vi "Tactile Controller v1.3.vi"() -> ()   [LabVIEW 2013]
uses:
  <vilib>/Instr/_visa.llb/VISA Configure Serial Port (Instr).vi
panel:
  in  "Refresh":bool
  in  "Switch":bool
  in  "Comm":bool
  out "Message Board":string
  in  "Serial Port":refnum<visa-resource-name>="COM7"
  in  "stop":bool
  out "read buffer":string
  in  "Trials":dbl=200.0
  in  "Inter-Stimulus Interval":dbl=1200.0
  in  "Vibro cycles":dbl=20.0
  in  "Jitter":dbl=100.0
  in  "Pin up duration":dbl=5.0
  in  "Stimuli Type":T1(ring)=enum."Steady State"
  in  "Cell5":bool=TRUE
  in  "Cell4":bool=TRUE
  in  "Cell3":bool=TRUE
  in  "Cell2":bool=TRUE
  in  "Cell1":bool=TRUE
  in  "SSF5":dbl=11.0
  in  "SSF4":dbl=8.0
  in  "SSF3":dbl=7.0
  in  "SSF2":dbl=5.0
  in  "SSF1":dbl=2.0
  in  "C5P8":bool=TRUE
  in  "C5P7":bool=TRUE
  in  "C5P6":bool=TRUE
  in  "C5P5":bool=TRUE
  in  "C5P4":bool=TRUE
  in  "C5P3":bool=TRUE
  in  "C5P2":bool=TRUE
  in  "C5P1":bool=TRUE
  in  "C4P8":bool=TRUE
  in  "C4P7":bool=TRUE
  in  "C4P6":bool=TRUE
  in  "C4P5":bool=TRUE
  in  "C4P4":bool=TRUE
  in  "C4P3":bool=TRUE
  in  "C4P2":bool=TRUE
  in  "C4P1":bool=TRUE
  in  "C3P8":bool=TRUE
  in  "C3P7":bool=TRUE
  in  "C3P6":bool=TRUE
  in  "C3P5":bool=TRUE
  in  "C3P4":bool=TRUE
  in  "C3P3":bool=TRUE
  in  "C3P2":bool=TRUE
  in  "C3P1":bool=TRUE
  in  "C2P8":bool=TRUE
  in  "C2P7":bool=TRUE
  in  "C2P6":bool=TRUE
  in  "C2P5":bool=TRUE
  in  "C2P4":bool=TRUE
  in  "C2P3":bool=TRUE
  in  "C2P2":bool=TRUE
  in  "C2P1":bool=TRUE
  in  "C1P8":bool=TRUE
  in  "C1P7":bool=TRUE
  in  "C1P6":bool=TRUE
  in  "C1P5":bool=TRUE
  in  "C1P4":bool=TRUE
  in  "C1P3":bool=TRUE
  in  "C1P2":bool=TRUE
  in  "C1P1":bool=TRUE
  # "ms"
  # "ms"
  # "ms"
  # "1                           2                         3                        4                         5"
  # "Steady State Frequency [Hz]"
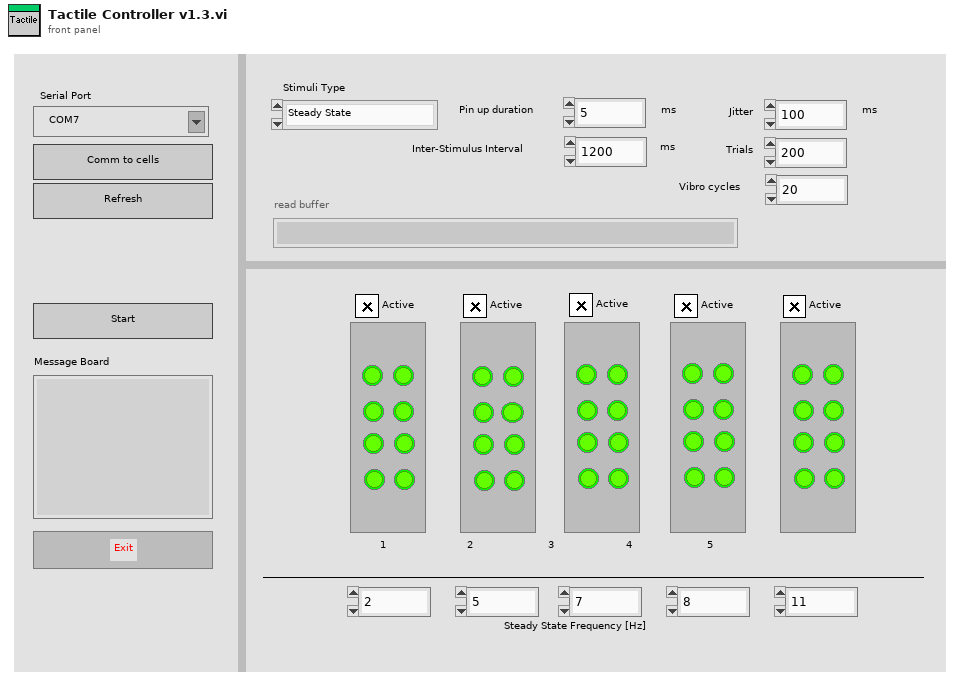
[diagram p1: front panel]
types:
  T1 = enum16{"Transient", "Steady State", "Vibrotactile"}
  T2 = enum8{"Enabled", "Disabled", "Disabled and Grayed Out"}
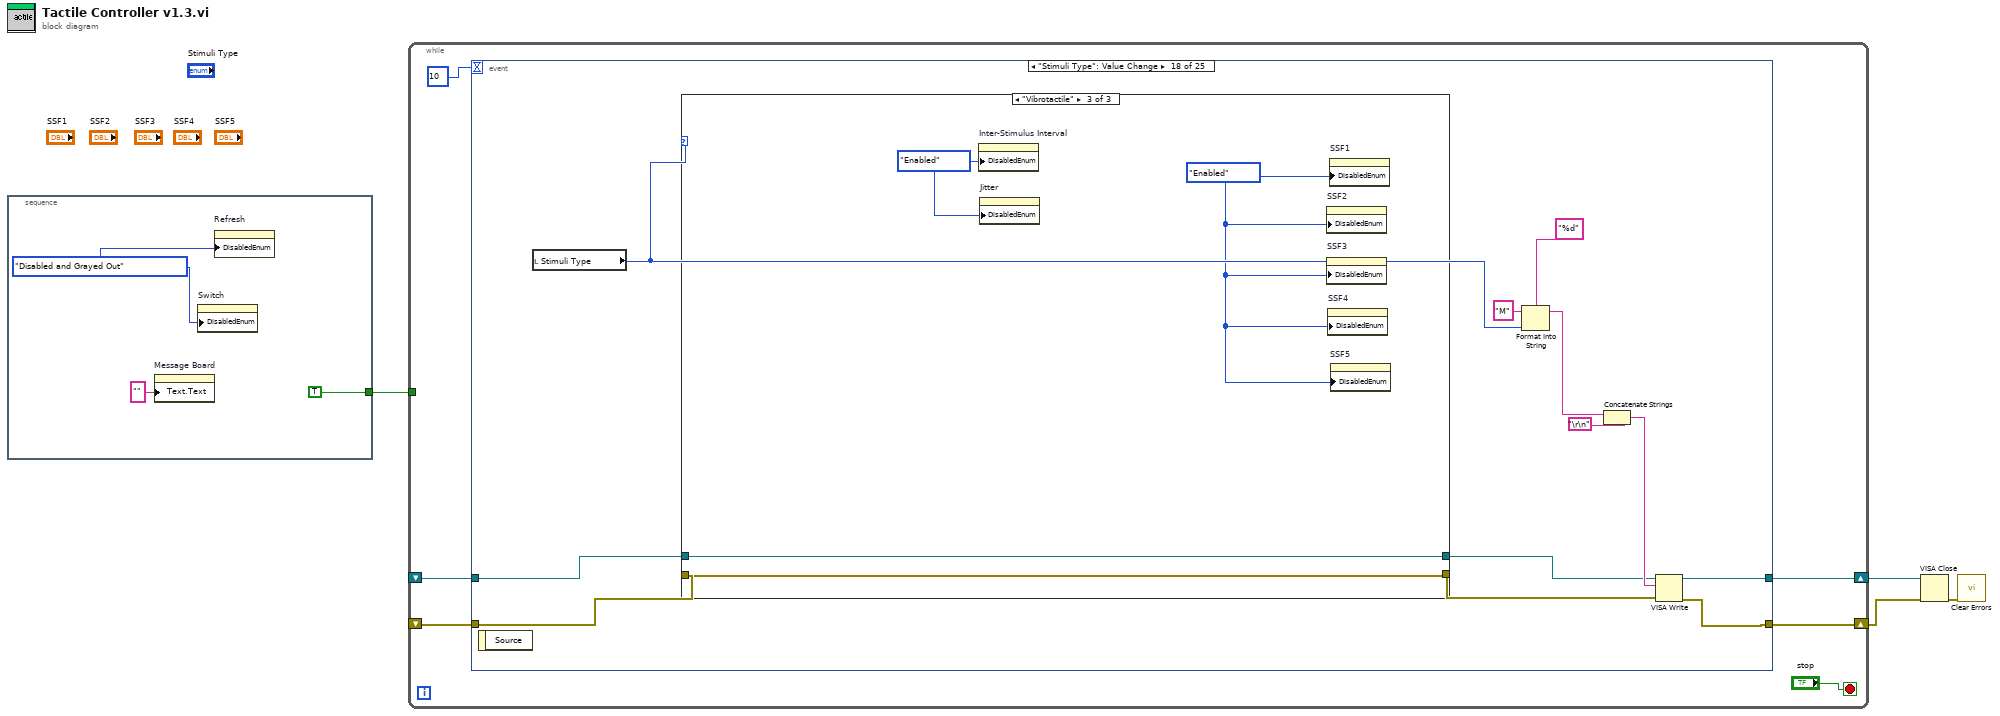
[diagram p0: block diagram]
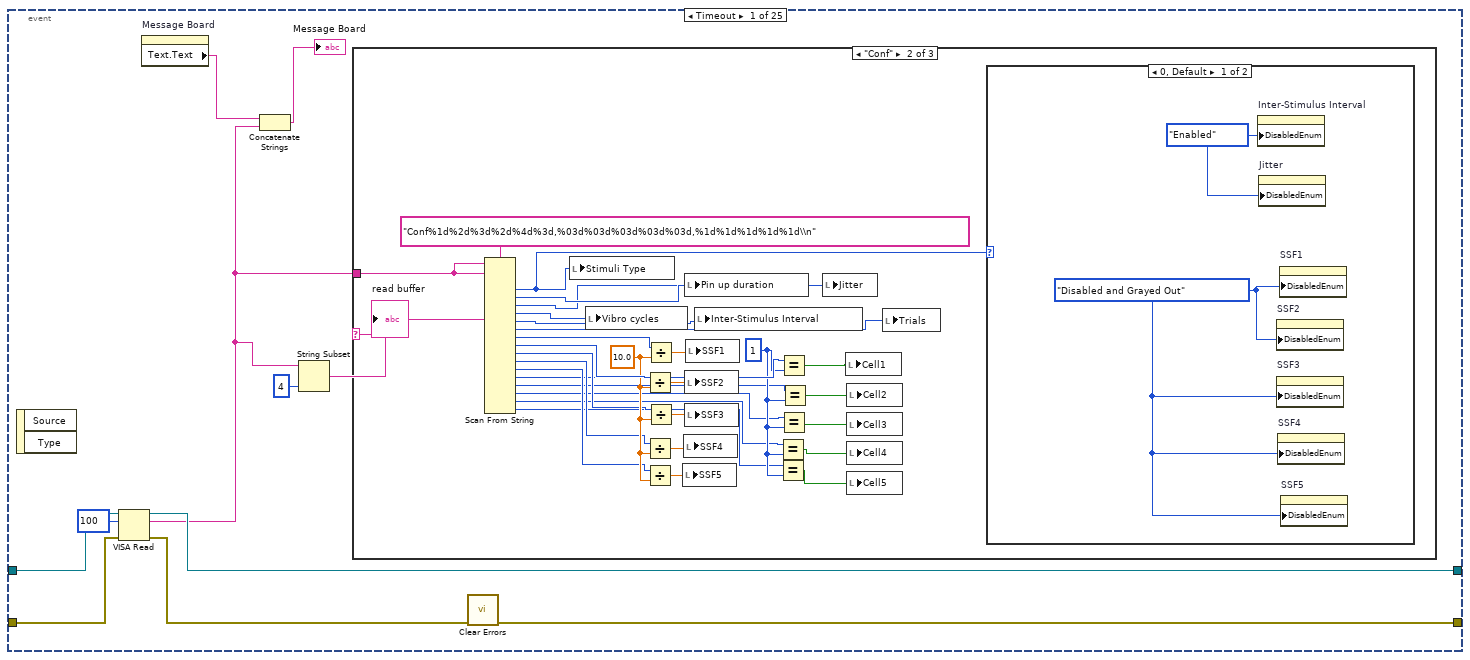
[diagram p2: hidden frame]
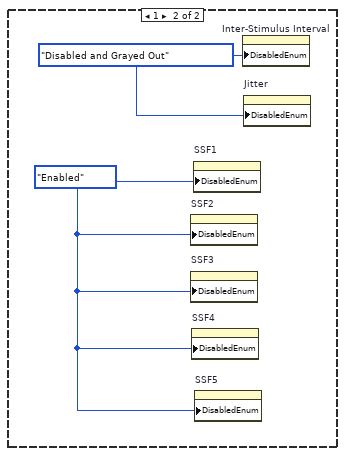
[diagram p4: hidden frame]
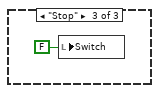
[diagram p5: hidden frame]
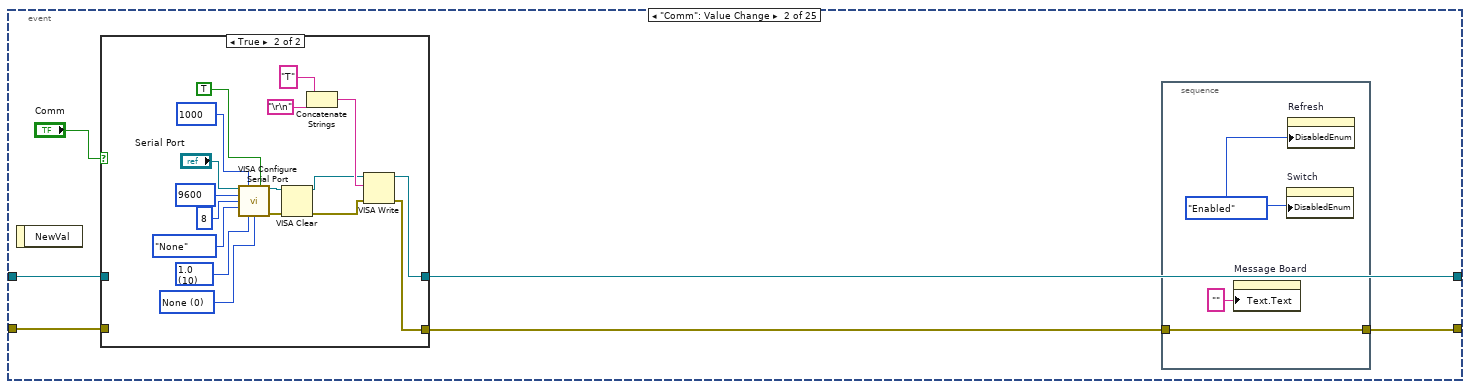
[diagram p6: hidden frame]
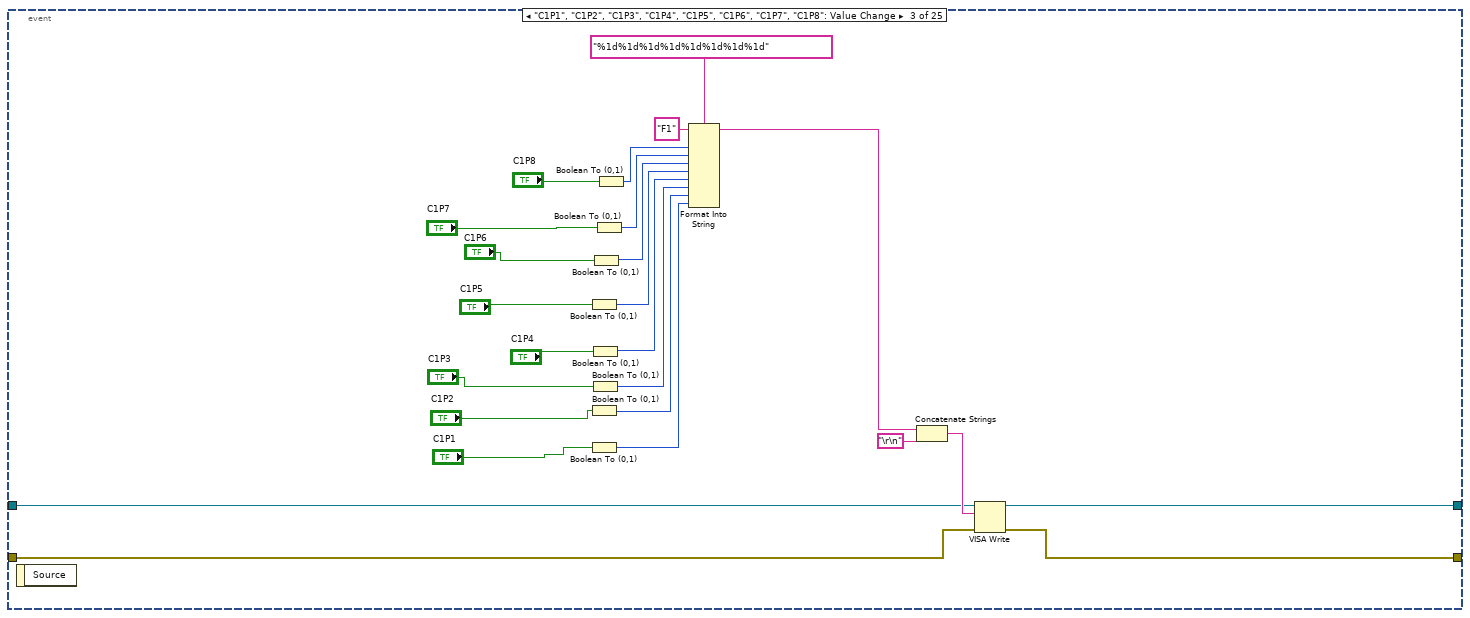
[diagram p8: hidden frame]
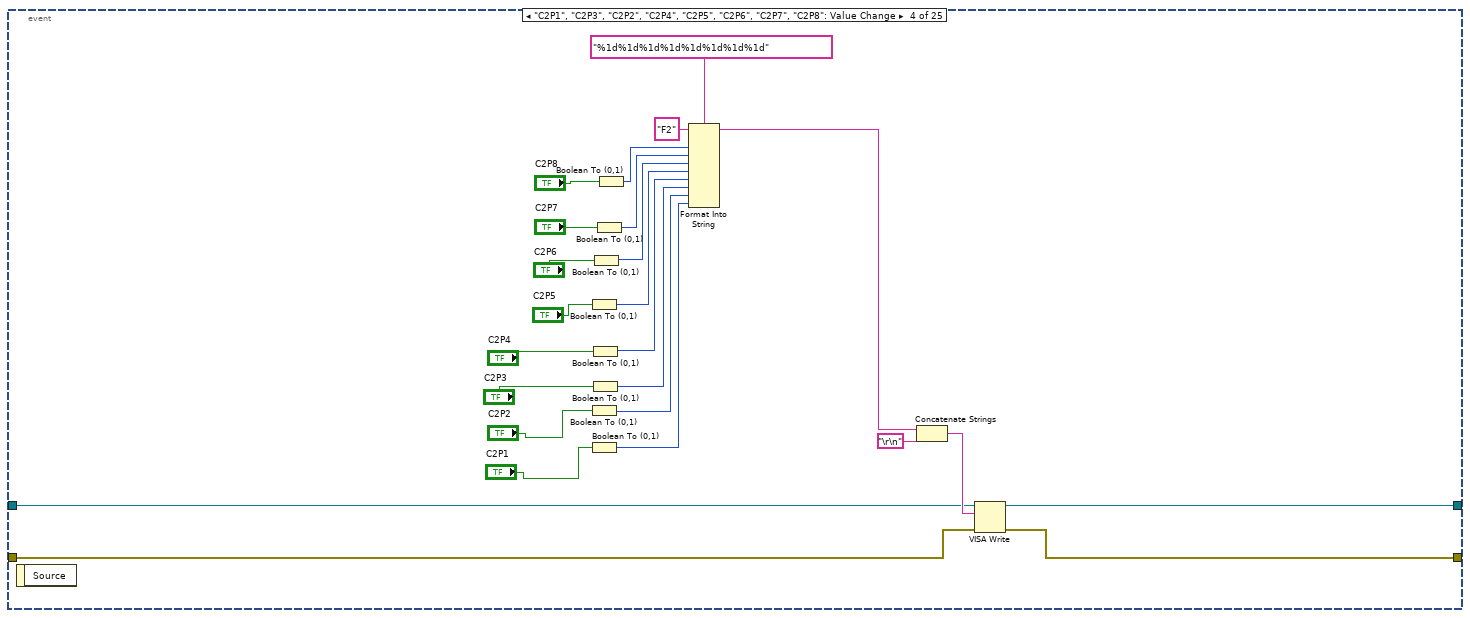
[diagram p9: hidden frame]
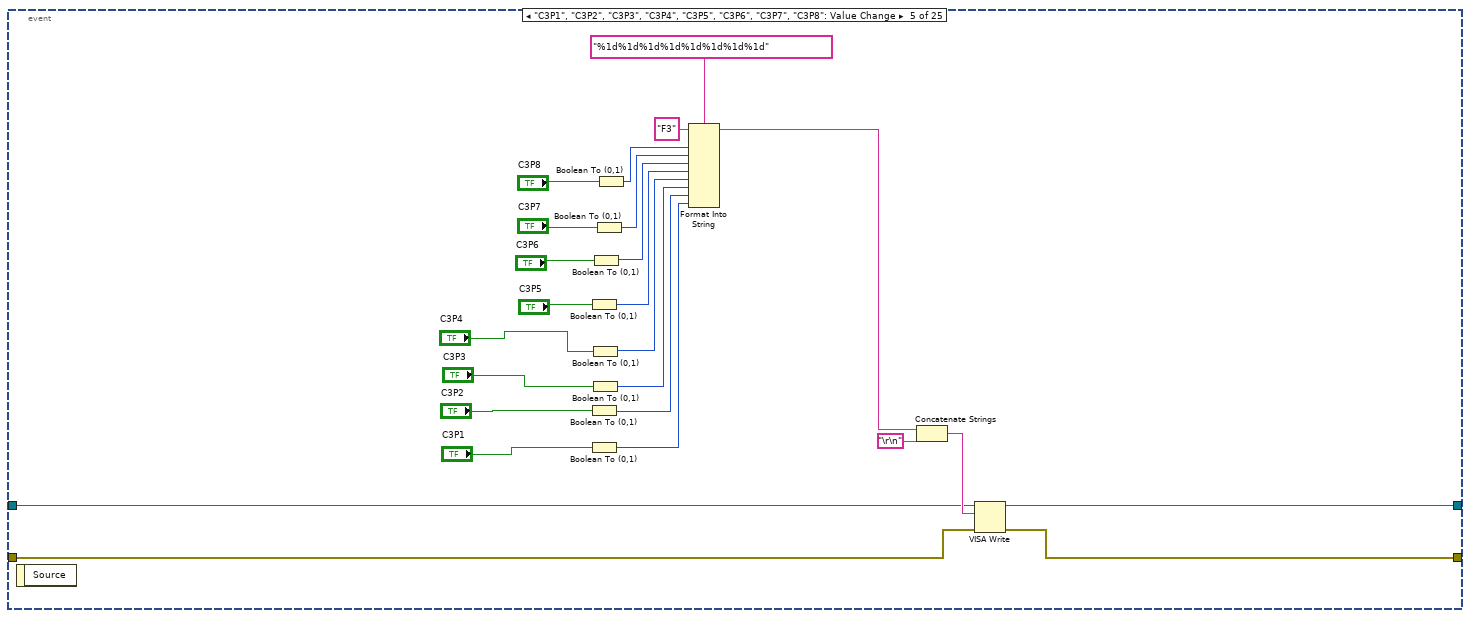
[diagram p10: hidden frame]
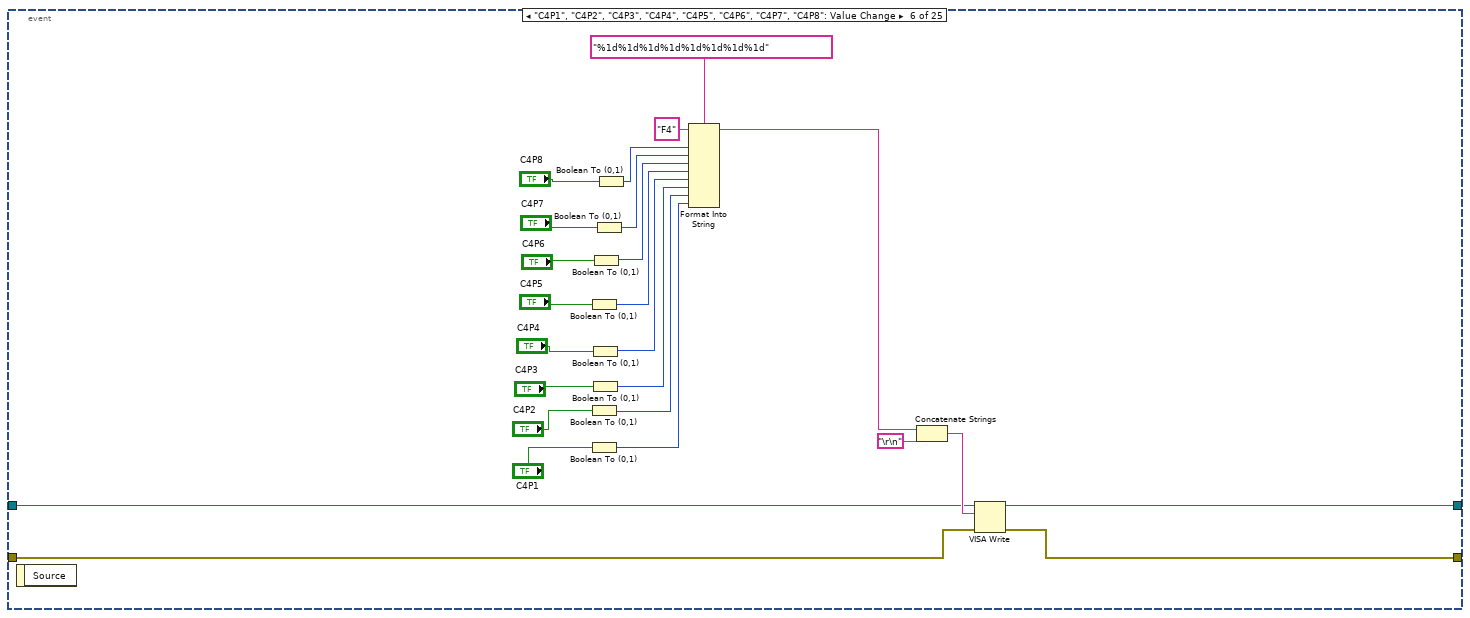
[diagram p11: hidden frame]
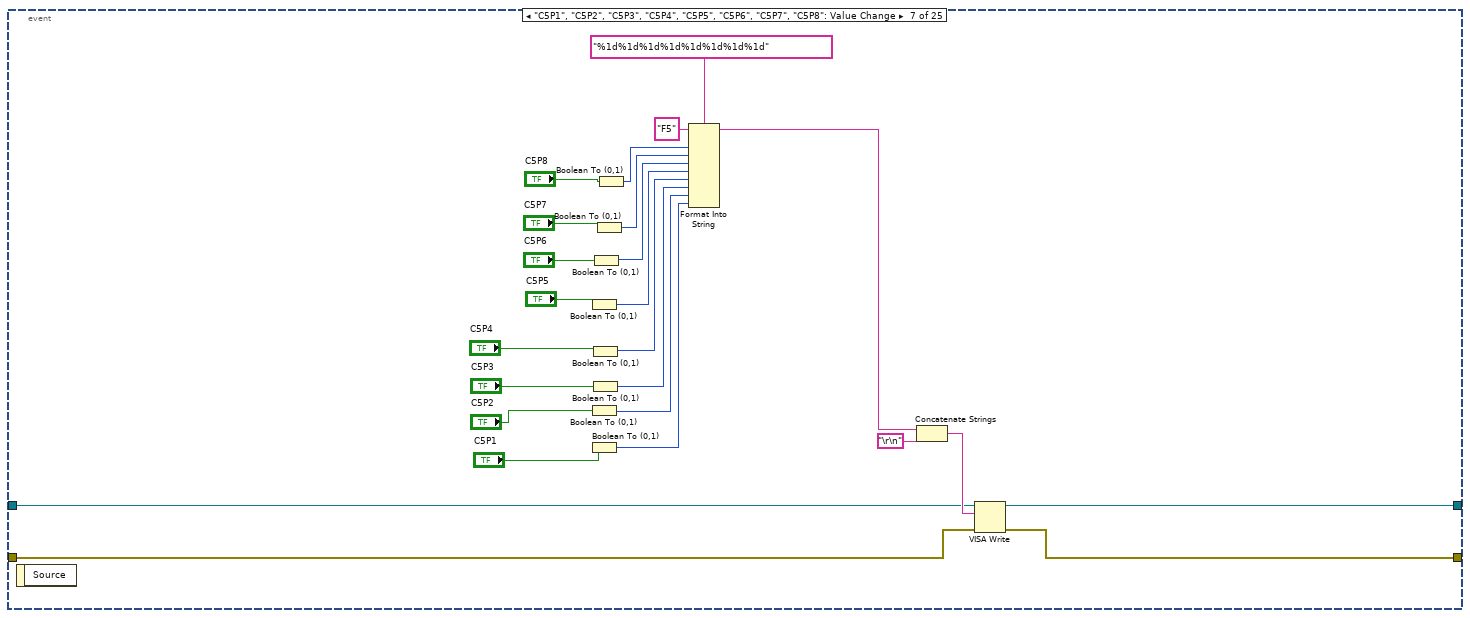
[diagram p12: hidden frame]
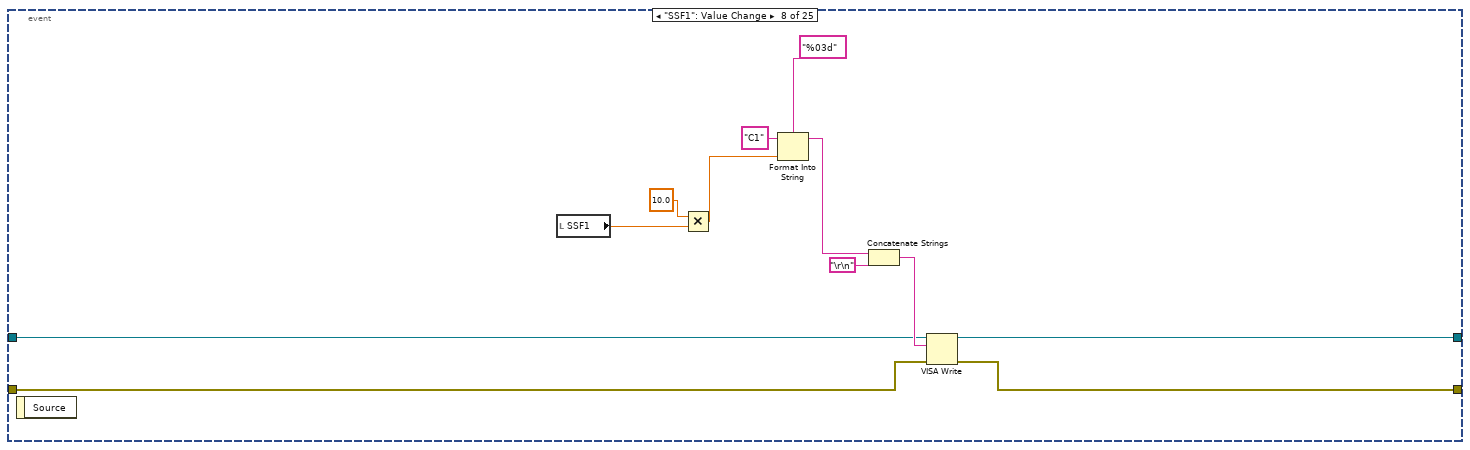
[diagram p13: hidden frame]
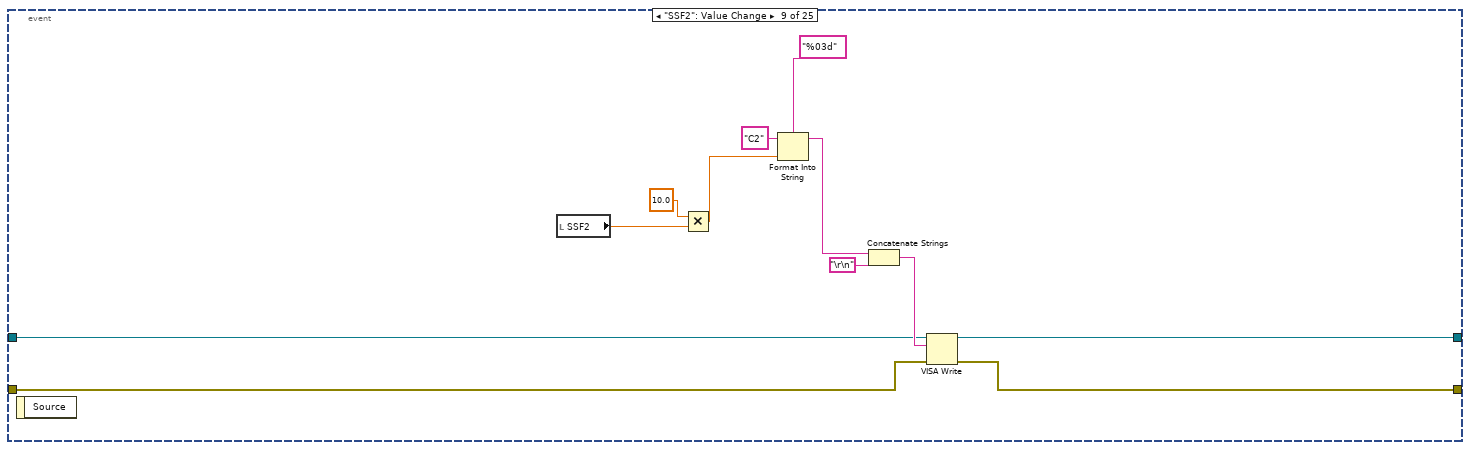
[diagram p14: hidden frame]
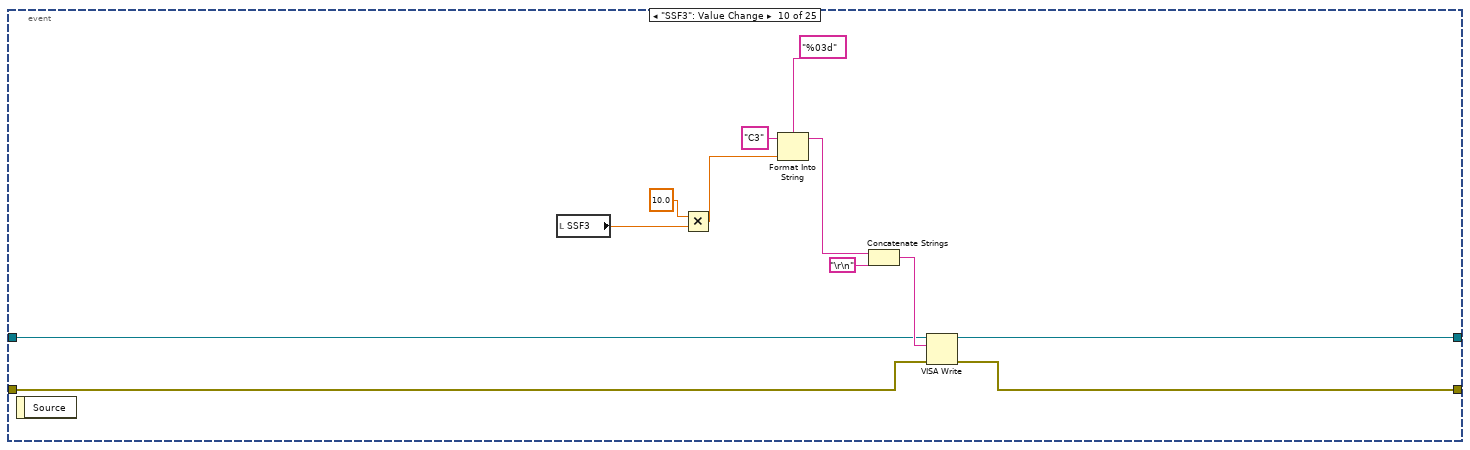
[diagram p15: hidden frame]
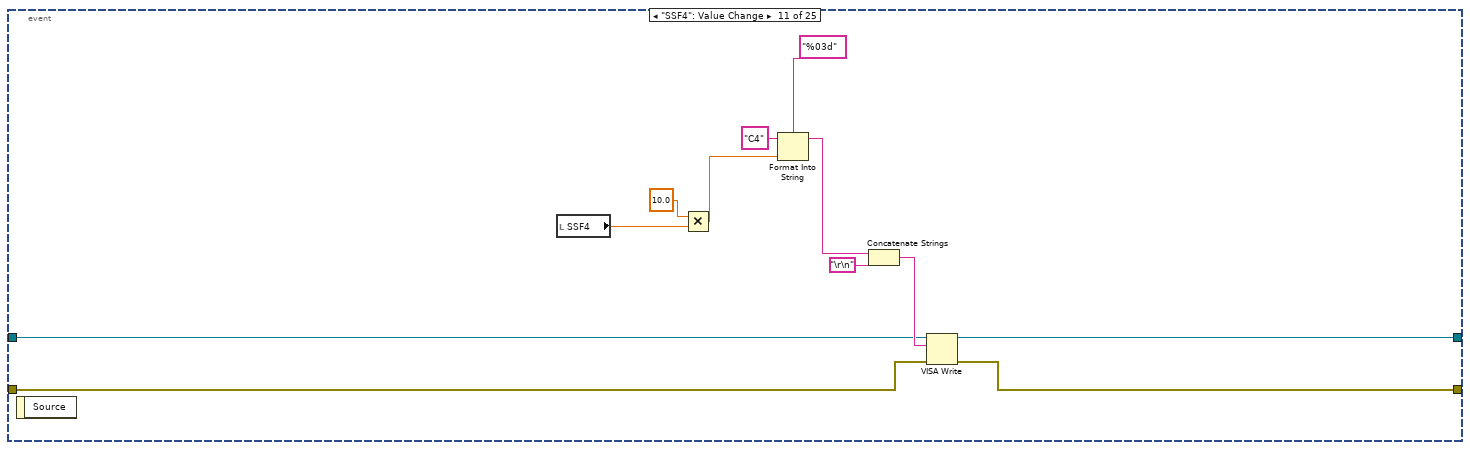
[diagram p16: hidden frame]
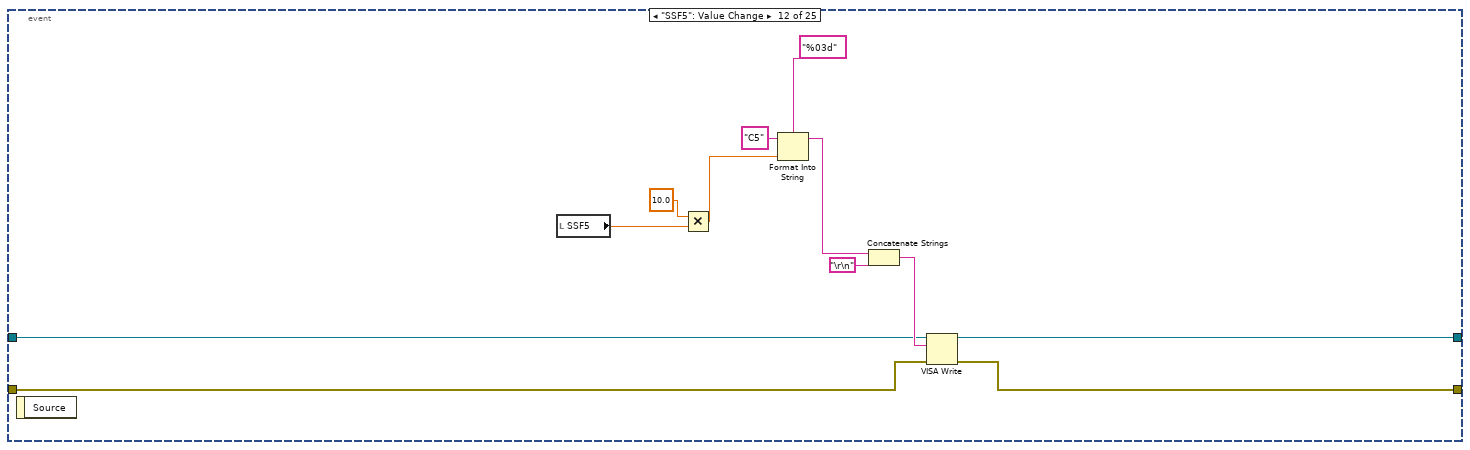
[diagram p17: hidden frame]
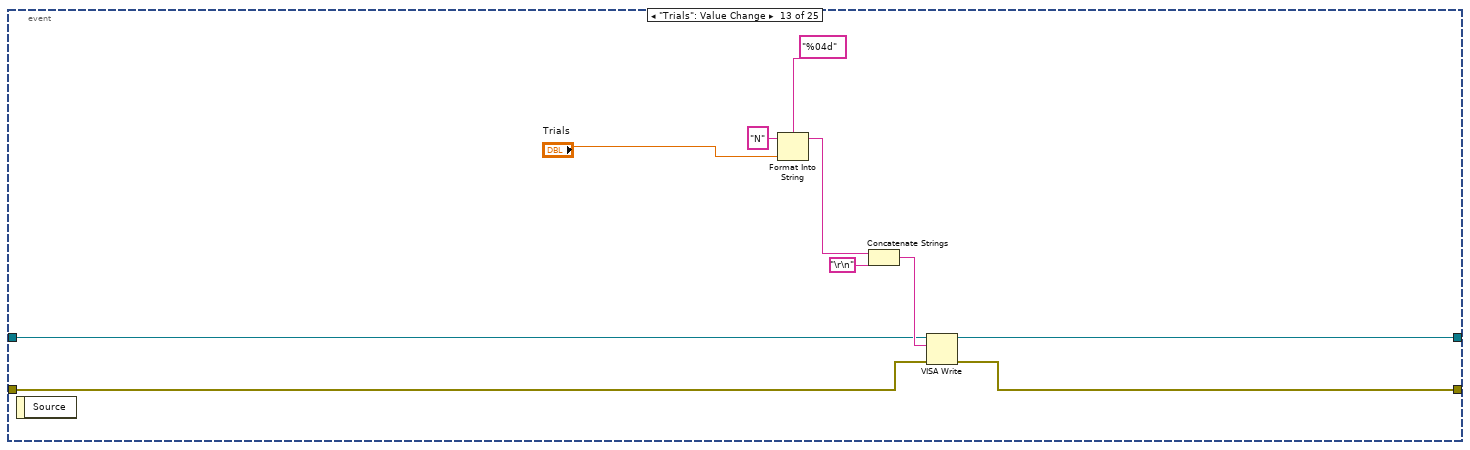
[diagram p18: hidden frame]
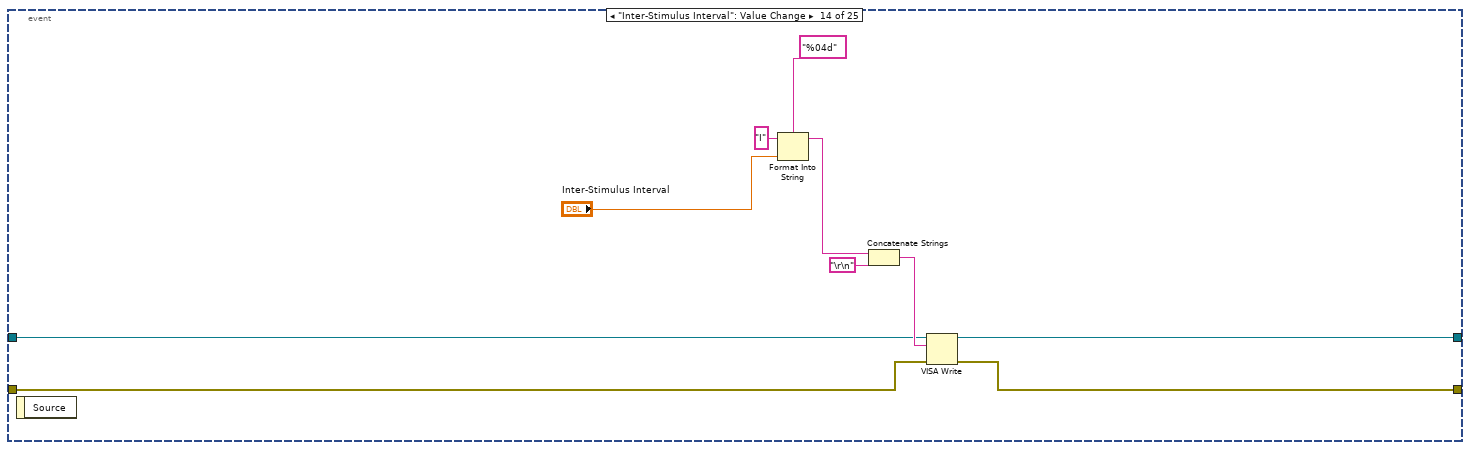
[diagram p19: hidden frame]
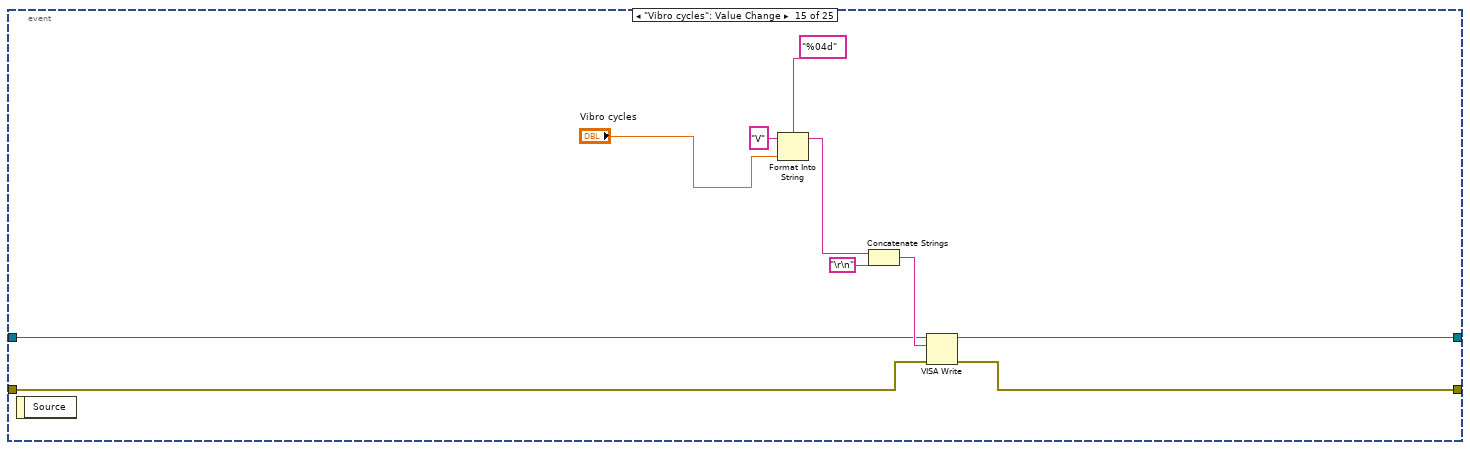
[diagram p20: hidden frame]
diagram:
  n1 = stacked-sequence {
    tunnel: [TRUE] -> w1
    frame #0 {
      w5 = T2."Disabled and Grayed Out" ("Disabled")
      n2 = property on="Message Board" class="Str"("Text.Text"="") -> ()  [unwired: 2 in, 2 out]
      n3 = property on="Switch" class="Bool (strict)"("DisabledEnum"=w5) -> ()  [unwired: 2 in, 2 out]
      n4 = property on="Refresh" class="Bool (strict)"("DisabledEnum"=w5) -> ()  [unwired: 2 in, 2 out]
    }
  }
  n5 = while {
    shift-right: [w11] -> w3
    shift-left: _ -> [w12]
    shift-right: [w8] -> w2
    shift-left: _ -> [w9]
    tunnel: w1 -> [_]
    stop <- "stop" stop-if-true
    n6 = event shown="[17] \"Stimuli Type\": Value Change" {
      selector: _ -> [_ _ _ _ _ _ _ _ _ _ _ _ _ _ _ _ _ _ _ _ _ _ _ _ _]
      dyn-events: _ -> [_ _ _ _ _ _ _ _ _ _ _ _ _ _ _ _ _ _ _ _ _ _ _ _ _]
      timeout: u32 10 ("milliseconds to wait") -> [_ _ _ _ _ _ _ _ _ _ _ _ _ _ _ _ _ _ _ _ _ _ _ _ _]
      tunnel: w12 -> [w22 w64 w98 w123 w148 w173 w198 w218 w230 w242 w254 w266 w276 w286 w296 w306 w316 w333 w349 w361 w372 w383 w394 w406 w423]
      tunnel: [w24 w62 w96 w121 w146 w171 w196 w216 w228 w240 w252 w264 w274 w284 w294 w304 w314 w323 w348 w360 w371 w382 w393 w405 w422] -> w11
      tunnel: w9 -> [w21 w63 w99 w124 w149 w174 w199 w219 w231 w243 w255 w267 w277 w287 w297 w307 w317 w334 w351 w363 w374 w385 w396 w404 w425]
      tunnel: [w20 w60 w97 w122 w147 w172 w197 w217 w229 w241 w253 w265 w275 w285 w295 w305 w315 w325 w347 w359 w370 w381 w392 w403 w424] -> w8
      event Timeout {
        n7 = event-data() -> ()  [unwired: 1 in, 2 out]
        n8 = VISA Read(VISA resource name=w21, byte count=u32 100, error in (no error)=w22) -> (VISA resource name out=w20:refnum<visa-resource-name>, read buffer=w14:string, error out=w19:errorcluster)  [unwired: 1 out]
        n9 = property on="Message Board" class="Str"() -> ("Text.Text"=w17:string)  [unwired: 2 in, 2 out]
        n10 = Concatenate Strings(w17, w14) -> (→"Message Board":string)
        n11 = String Subset(string=w14, length (rest)=4 ("length (rest)")) -> (substring=w15:string)  [unwired: 1 in]
        n12 = case shown="\"Conf\"" w15 {
          tunnel: w14 -> [_ w54 _]
          frame Default {
          }
          frame "Conf" {
            w34 = i8 1 ("y")
            w42 = 10.0 ("y")
            n13 = Scan From String(format string="Conf%1d%2d%3d%2d%4d%3d,%03d%03d%03d%03d%03d,%1d%1d%1d%1d%1d\\n", input string=w54) -> (output 1=w25:i32, output 2=w52:i32, output 3=w51:i32, output 4=w50:i32, output 5=w49:i32, output 6=w48:i32, output 7=w47:i32, output 8=w44:i32, output 9=w41:i32, output 10=w40:i32, output 11=w39:i32, output 12=w36:i32, output 13=w33:i32, output 14=w32:i32, output 15=w31:i32, output 16=w30:i32)  [unwired: 18 in, 3 out]
            n14 = local write "Stimuli Type"(w25) -> ()
            n15 = local write "Vibro cycles"(w50) -> ()
            n16 = Divide(x=w44, y=w42) -> (x/y=w45:dbl)
            n17 = Divide(x=w40, y=w42) -> (x/y=w38:dbl)
            n18 = Divide(x=w39, y=w42) -> (x/y=w37:dbl)
            n19 = Divide(x=w47, y=w42) -> (x/y=w46:dbl)
            n20 = Divide(x=w41, y=w42) -> (x/y=w43:dbl)
            n21 = local write "SSF5"(w37) -> ()
            n22 = local write "SSF4"(w38) -> ()
            n23 = local write "Pin up duration"(w52) -> ()
            n24 = local write "SSF2"(w45) -> ()
            n25 = local write "SSF3"(w43) -> ()
            n26 = local write "SSF1"(w46) -> ()
            n27 = local write "Inter-Stimulus Interval"(w49) -> ()
            n28 = Equal?(x=w31, y=w34) -> (x = y?=w27:bool)
            n29 = Equal?(x=w30, y=w34) -> (x = y?=w26:bool)
            n30 = Equal?(x=w36, y=w34) -> (x = y?=w35:bool)
            n31 = Equal?(x=w32, y=w34) -> (x = y?=w28:bool)
            n32 = Equal?(x=w33, y=w34) -> (x = y?=w29:bool)
            n33 = local write "Jitter"(w51) -> ()
            n34 = local write "Cell1"(w35) -> ()
            n35 = local write "Cell2"(w29) -> ()
            n36 = local write "Cell3"(w28) -> ()
            n37 = local write "Cell4"(w27) -> ()
            n38 = local write "Cell5"(w26) -> ()
            n39 = local write "Trials"(w48) -> ()
            n40 = case shown="0, Default" w25 {
              frame 0, Default {
                w55 = T2."Enabled" ("Disabled")
                w56 = T2."Disabled and Grayed Out" ("Disabled")
                n41 = property on="Inter-Stimulus Interval" class="DigNum (strict)"("DisabledEnum"=w55) -> ()  [unwired: 2 in, 2 out]
                n42 = property on="Jitter" class="DigNum (strict)"("DisabledEnum"=w55) -> ()  [unwired: 2 in, 2 out]
                n43 = property on="SSF2" class="DigNum (strict)"("DisabledEnum"=w56) -> ()  [unwired: 2 in, 2 out]
                n44 = property on="SSF3" class="DigNum (strict)"("DisabledEnum"=w56) -> ()  [unwired: 2 in, 2 out]
                n45 = property on="SSF4" class="DigNum (strict)"("DisabledEnum"=w56) -> ()  [unwired: 2 in, 2 out]
                n46 = property on="SSF1" class="DigNum (strict)"("DisabledEnum"=w56) -> ()  [unwired: 2 in, 2 out]
                n47 = property on="SSF5" class="DigNum (strict)"("DisabledEnum"=w56) -> ()  [unwired: 2 in, 2 out]
              }
              frame 1 {
                w57 = T2."Enabled" ("Disabled")
                w58 = T2."Disabled and Grayed Out" ("Disabled")
                n48 = property on="SSF2" class="DigNum (strict)"("DisabledEnum"=w57) -> ()  [unwired: 2 in, 2 out]
                n49 = property on="SSF3" class="DigNum (strict)"("DisabledEnum"=w57) -> ()  [unwired: 2 in, 2 out]
                n50 = property on="SSF4" class="DigNum (strict)"("DisabledEnum"=w57) -> ()  [unwired: 2 in, 2 out]
                n51 = property on="SSF1" class="DigNum (strict)"("DisabledEnum"=w57) -> ()  [unwired: 2 in, 2 out]
                n52 = property on="SSF5" class="DigNum (strict)"("DisabledEnum"=w57) -> ()  [unwired: 2 in, 2 out]
                n53 = property on="Inter-Stimulus Interval" class="DigNum (strict)"("DisabledEnum"=w58) -> ()  [unwired: 2 in, 2 out]
                n54 = property on="Jitter" class="DigNum (strict)"("DisabledEnum"=w58) -> ()  [unwired: 2 in, 2 out]
              }
            }
            "read buffer" <- w54
          }
          frame "Stop" {
            n55 = local write "Switch"(FALSE ("Switch")) -> ()
          }
        }
        n56 = call <vilib>:"Clear Errors.vi"("error in (no error)"=w19) -> ("error out"=w24:errorcluster)  [unwired: 6 in]
      }
      event "Comm": Value Change {
        n57 = event-data() -> ()  [unwired: 1 in, 1 out]
        n58 = case shown="True" "Comm" {
          tunnel: [w69 w71] -> w60
          tunnel: [w70 w72] -> w61
          tunnel: w64 -> [w70 _]
          tunnel: w63 -> [w69 _]
          frame False {
          }
          frame True {
            w80 = u16 0 items=["None", "XON/XOFF", "RTS/CTS", "XON/XOFF & RTS/CTS", "DTR/DSR", "XON/XOFF & DTR/DSR"] ("flow control (0:none)")
            w79 = u16 10 items=["1.0"=10, "1.5"=15, "2.0"=20] ("stop bits (10: 1 bit)")
            n59 = call-poly "VISA Configure Serial Port"("VISA resource name"="Serial Port", "timeout (10sec)"=u32 1000, "Enable Termination\nChar (T)"=TRUE ("Enable Termination\nChar (T)"), "baud rate (9600)"=u32 9600, "data bits (8)"=u16 8, "parity (0:none)"=enum16{"None", "Odd", "Even", "Mark", "Space"}."None", "stop bits (10: 1 bit)"=w79, "flow control (0:none)"=w80) -> ("VISA resource name out"=w81:refnum<visa-resource-name>, "error out"=w82:errorcluster)  [unwired: 6 in]
            n60 = VISA Clear(VISA resource name=w81, error in (no error)=w82) -> (VISA resource name out=w83:refnum<visa-resource-name>, error out=w84:errorcluster)
            n61 = Concatenate Strings("T" ("write buffer"), "\r\n") -> (w87:string)
            n62 = VISA Write(VISA resource name=w83, write buffer=w87, error in (no error)=w84) -> (VISA resource name out=w71:refnum<visa-resource-name>, error out=w72:errorcluster)  [unwired: 1 out]
          }
        }
        n63 = stacked-sequence {
          tunnel: w61 -> [w68]
          tunnel: [w68] -> w62
          frame #0 {
            w66 = T2."Enabled" ("Disabled")
            n64 = property on="Message Board" class="Str"("Text.Text"="") -> ()  [unwired: 2 in, 2 out]
            n65 = property on="Switch" class="Bool (strict)"("DisabledEnum"=w66) -> ()  [unwired: 2 in, 2 out]
            n66 = property on="Refresh" class="Bool (strict)"("DisabledEnum"=w66) -> ()  [unwired: 2 in, 2 out]
          }
        }
      }
      event "C1P1", "C1P2", "C1P3", "C1P4", "C1P5", "C1P6", "C1P7", "C1P8": Value Change {
        n67 = event-data() -> ()  [unwired: 1 in, 1 out]
        n68 = Boolean To (0,1)(Boolean="C1P5") -> (0, 1=w108:i16)
        n69 = Boolean To (0,1)(Boolean="C1P2") -> (0, 1=w105:i16)
        n70 = Boolean To (0,1)(Boolean="C1P1") -> (0, 1=w104:i16)
        n71 = Boolean To (0,1)(Boolean="C1P4") -> (0, 1=w107:i16)
        n72 = Boolean To (0,1)(Boolean="C1P3") -> (0, 1=w106:i16)
        n73 = Boolean To (0,1)(Boolean="C1P6") -> (0, 1=w109:i16)
        n74 = Boolean To (0,1)(Boolean="C1P7") -> (0, 1=w110:i16)
        n75 = Boolean To (0,1)(Boolean="C1P8") -> (0, 1=w112:i16)
        n76 = Format Into String(format string="%1d%1d%1d%1d%1d%1d%1d%1d", initial string="F1", w112, w110, w109, w108, w107, w106, w105, w104) -> (resulting string=w100:string)  [unwired: 1 in, 1 out]
        n77 = Concatenate Strings(w100, "\r\n") -> (w101:string)
        n78 = VISA Write(VISA resource name=w99, write buffer=w101, error in (no error)=w98) -> (VISA resource name out=w97:refnum<visa-resource-name>, error out=w96:errorcluster)  [unwired: 1 out]
      }
      event "C2P1", "C2P3", "C2P2", "C2P4", "C2P5", "C2P6", "C2P7", "C2P8": Value Change {
        n79 = event-data() -> ()  [unwired: 1 in, 1 out]
        n80 = Boolean To (0,1)(Boolean="C2P5") -> (0, 1=w133:i16)
        n81 = Boolean To (0,1)(Boolean="C2P2") -> (0, 1=w130:i16)
        n82 = Boolean To (0,1)(Boolean="C2P1") -> (0, 1=w129:i16)
        n83 = Boolean To (0,1)(Boolean="C2P4") -> (0, 1=w132:i16)
        n84 = Boolean To (0,1)(Boolean="C2P3") -> (0, 1=w131:i16)
        n85 = Boolean To (0,1)(Boolean="C2P6") -> (0, 1=w134:i16)
        n86 = Boolean To (0,1)(Boolean="C2P7") -> (0, 1=w135:i16)
        n87 = Boolean To (0,1)(Boolean="C2P8") -> (0, 1=w137:i16)
        n88 = Format Into String(format string="%1d%1d%1d%1d%1d%1d%1d%1d", initial string="F2", w137, w135, w134, w133, w132, w131, w130, w129) -> (resulting string=w125:string)  [unwired: 1 in, 1 out]
        n89 = Concatenate Strings(w125, "\r\n") -> (w126:string)
        n90 = VISA Write(VISA resource name=w124, write buffer=w126, error in (no error)=w123) -> (VISA resource name out=w122:refnum<visa-resource-name>, error out=w121:errorcluster)  [unwired: 1 out]
      }
      event "C3P1", "C3P2", "C3P3", "C3P4", "C3P5", "C3P6", "C3P7", "C3P8": Value Change {
        n91 = event-data() -> ()  [unwired: 1 in, 1 out]
        n92 = Boolean To (0,1)(Boolean="C3P5") -> (0, 1=w158:i16)
        n93 = Boolean To (0,1)(Boolean="C3P2") -> (0, 1=w155:i16)
        n94 = Boolean To (0,1)(Boolean="C3P1") -> (0, 1=w154:i16)
        n95 = Boolean To (0,1)(Boolean="C3P4") -> (0, 1=w157:i16)
        n96 = Boolean To (0,1)(Boolean="C3P3") -> (0, 1=w156:i16)
        n97 = Boolean To (0,1)(Boolean="C3P6") -> (0, 1=w159:i16)
        n98 = Boolean To (0,1)(Boolean="C3P7") -> (0, 1=w160:i16)
        n99 = Boolean To (0,1)(Boolean="C3P8") -> (0, 1=w162:i16)
        n100 = Format Into String(format string="%1d%1d%1d%1d%1d%1d%1d%1d", initial string="F3", w162, w160, w159, w158, w157, w156, w155, w154) -> (resulting string=w150:string)  [unwired: 1 in, 1 out]
        n101 = Concatenate Strings(w150, "\r\n") -> (w151:string)
        n102 = VISA Write(VISA resource name=w149, write buffer=w151, error in (no error)=w148) -> (VISA resource name out=w147:refnum<visa-resource-name>, error out=w146:errorcluster)  [unwired: 1 out]
      }
      event "C4P1", "C4P2", "C4P3", "C4P4", "C4P5", "C4P6", "C4P7", "C4P8": Value Change {
        n103 = event-data() -> ()  [unwired: 1 in, 1 out]
        n104 = Boolean To (0,1)(Boolean="C4P5") -> (0, 1=w183:i16)
        n105 = Boolean To (0,1)(Boolean="C4P2") -> (0, 1=w180:i16)
        n106 = Boolean To (0,1)(Boolean="C4P1") -> (0, 1=w179:i16)
        n107 = Boolean To (0,1)(Boolean="C4P4") -> (0, 1=w182:i16)
        n108 = Boolean To (0,1)(Boolean="C4P3") -> (0, 1=w181:i16)
        n109 = Boolean To (0,1)(Boolean="C4P6") -> (0, 1=w184:i16)
        n110 = Boolean To (0,1)(Boolean="C4P7") -> (0, 1=w185:i16)
        n111 = Boolean To (0,1)(Boolean="C4P8") -> (0, 1=w187:i16)
        n112 = Format Into String(format string="%1d%1d%1d%1d%1d%1d%1d%1d", initial string="F4", w187, w185, w184, w183, w182, w181, w180, w179) -> (resulting string=w175:string)  [unwired: 1 in, 1 out]
        n113 = Concatenate Strings(w175, "\r\n") -> (w176:string)
        n114 = VISA Write(VISA resource name=w174, write buffer=w176, error in (no error)=w173) -> (VISA resource name out=w172:refnum<visa-resource-name>, error out=w171:errorcluster)  [unwired: 1 out]
      }
      event "C5P1", "C5P2", "C5P3", "C5P4", "C5P5", "C5P6", "C5P7", "C5P8": Value Change {
        n115 = event-data() -> ()  [unwired: 1 in, 1 out]
        n116 = Boolean To (0,1)(Boolean="C5P5") -> (0, 1=w208:i16)
        n117 = Boolean To (0,1)(Boolean="C5P2") -> (0, 1=w205:i16)
        n118 = Boolean To (0,1)(Boolean="C5P1") -> (0, 1=w204:i16)
        n119 = Boolean To (0,1)(Boolean="C5P4") -> (0, 1=w207:i16)
        n120 = Boolean To (0,1)(Boolean="C5P3") -> (0, 1=w206:i16)
        n121 = Boolean To (0,1)(Boolean="C5P6") -> (0, 1=w209:i16)
        n122 = Boolean To (0,1)(Boolean="C5P7") -> (0, 1=w210:i16)
        n123 = Boolean To (0,1)(Boolean="C5P8") -> (0, 1=w212:i16)
        n124 = Format Into String(format string="%1d%1d%1d%1d%1d%1d%1d%1d", initial string="F5", w212, w210, w209, w208, w207, w206, w205, w204) -> (resulting string=w200:string)  [unwired: 1 in, 1 out]
        n125 = Concatenate Strings(w200, "\r\n") -> (w201:string)
        n126 = VISA Write(VISA resource name=w199, write buffer=w201, error in (no error)=w198) -> (VISA resource name out=w197:refnum<visa-resource-name>, error out=w196:errorcluster)  [unwired: 1 out]
      }
      event "SSF1": Value Change {
        n127 = event-data() -> ()  [unwired: 1 in, 1 out]
        n128 = local read "SSF1"() -> (w214:dbl)
        n129 = Multiply(x=10.0, y=w214) -> (x*y=w213:dbl)
        n130 = Format Into String(format string="%03d", initial string="C1", w213) -> (resulting string=w220:string)  [unwired: 1 in, 1 out]
        n131 = Concatenate Strings(w220, "\r\n") -> (w221:string)
        n132 = VISA Write(VISA resource name=w219, write buffer=w221, error in (no error)=w218) -> (VISA resource name out=w217:refnum<visa-resource-name>, error out=w216:errorcluster)  [unwired: 1 out]
      }
      event "SSF2": Value Change {
        n133 = event-data() -> ()  [unwired: 1 in, 1 out]
        n134 = local read "SSF2"() -> (w226:dbl)
        n135 = Multiply(x=10.0, y=w226) -> (x*y=w225:dbl)
        n136 = Format Into String(format string="%03d", initial string="C2", w225) -> (resulting string=w232:string)  [unwired: 1 in, 1 out]
        n137 = Concatenate Strings(w232, "\r\n") -> (w233:string)
        n138 = VISA Write(VISA resource name=w231, write buffer=w233, error in (no error)=w230) -> (VISA resource name out=w229:refnum<visa-resource-name>, error out=w228:errorcluster)  [unwired: 1 out]
      }
      event "SSF3": Value Change {
        n139 = event-data() -> ()  [unwired: 1 in, 1 out]
        n140 = local read "SSF3"() -> (w238:dbl)
        n141 = Multiply(x=10.0, y=w238) -> (x*y=w237:dbl)
        n142 = Format Into String(format string="%03d", initial string="C3", w237) -> (resulting string=w244:string)  [unwired: 1 in, 1 out]
        n143 = Concatenate Strings(w244, "\r\n") -> (w245:string)
        n144 = VISA Write(VISA resource name=w243, write buffer=w245, error in (no error)=w242) -> (VISA resource name out=w241:refnum<visa-resource-name>, error out=w240:errorcluster)  [unwired: 1 out]
      }
      event "SSF4": Value Change {
        n145 = event-data() -> ()  [unwired: 1 in, 1 out]
        n146 = local read "SSF4"() -> (w250:dbl)
        n147 = Multiply(x=10.0, y=w250) -> (x*y=w249:dbl)
        n148 = Format Into String(format string="%03d", initial string="C4", w249) -> (resulting string=w256:string)  [unwired: 1 in, 1 out]
        n149 = Concatenate Strings(w256, "\r\n") -> (w257:string)
        n150 = VISA Write(VISA resource name=w255, write buffer=w257, error in (no error)=w254) -> (VISA resource name out=w253:refnum<visa-resource-name>, error out=w252:errorcluster)  [unwired: 1 out]
      }
      event "SSF5": Value Change {
        n151 = event-data() -> ()  [unwired: 1 in, 1 out]
        n152 = local read "SSF5"() -> (w262:dbl)
        n153 = Multiply(x=10.0, y=w262) -> (x*y=w261:dbl)
        n154 = Format Into String(format string="%03d", initial string="C5", w261) -> (resulting string=w268:string)  [unwired: 1 in, 1 out]
        n155 = Concatenate Strings(w268, "\r\n") -> (w269:string)
        n156 = VISA Write(VISA resource name=w267, write buffer=w269, error in (no error)=w266) -> (VISA resource name out=w265:refnum<visa-resource-name>, error out=w264:errorcluster)  [unwired: 1 out]
      }
      event "Trials": Value Change {
        n157 = event-data() -> ()  [unwired: 1 in, 1 out]
        n158 = Format Into String(format string="%04d", initial string="N", "Trials") -> (resulting string=w278:string)  [unwired: 1 in, 1 out]
        n159 = Concatenate Strings(w278, "\r\n") -> (w279:string)
        n160 = VISA Write(VISA resource name=w277, write buffer=w279, error in (no error)=w276) -> (VISA resource name out=w275:refnum<visa-resource-name>, error out=w274:errorcluster)  [unwired: 1 out]
      }
      event "Inter-Stimulus Interval": Value Change {
        n161 = event-data() -> ()  [unwired: 1 in, 1 out]
        n162 = Format Into String(format string="%04d", initial string="I", "Inter-Stimulus Interval") -> (resulting string=w288:string)  [unwired: 1 in, 1 out]
        n163 = Concatenate Strings(w288, "\r\n") -> (w289:string)
        n164 = VISA Write(VISA resource name=w287, write buffer=w289, error in (no error)=w286) -> (VISA resource name out=w285:refnum<visa-resource-name>, error out=w284:errorcluster)  [unwired: 1 out]
      }
      event "Vibro cycles": Value Change {
        n165 = event-data() -> ()  [unwired: 1 in, 1 out]
        n166 = Format Into String(format string="%04d", initial string="V", "Vibro cycles") -> (resulting string=w298:string)  [unwired: 1 in, 1 out]
        n167 = Concatenate Strings(w298, "\r\n") -> (w299:string)
        n168 = VISA Write(VISA resource name=w297, write buffer=w299, error in (no error)=w296) -> (VISA resource name out=w295:refnum<visa-resource-name>, error out=w294:errorcluster)  [unwired: 1 out]
      }
      event "Jitter": Value Change {
        n169 = event-data() -> ()  [unwired: 1 in, 1 out]
        n170 = Format Into String(format string="%04d", initial string="J", "Jitter") -> (resulting string=w308:string)  [unwired: 1 in, 1 out]
        n171 = Concatenate Strings(w308, "\r\n") -> (w309:string)
        n172 = VISA Write(VISA resource name=w307, write buffer=w309, error in (no error)=w306) -> (VISA resource name out=w305:refnum<visa-resource-name>, error out=w304:errorcluster)  [unwired: 1 out]
      }
      event "Pin up duration": Value Change {
        n173 = event-data() -> ()  [unwired: 1 in, 1 out]
        n174 = Format Into String(format string="%03d", initial string="P", "Pin up duration") -> (resulting string=w318:string)  [unwired: 1 in, 1 out]
        n175 = Concatenate Strings(w318, "\r\n") -> (w319:string)
        n176 = VISA Write(VISA resource name=w317, write buffer=w319, error in (no error)=w316) -> (VISA resource name out=w315:refnum<visa-resource-name>, error out=w314:errorcluster)  [unwired: 1 out]
      }
      event "Stimuli Type": Value Change {
        n177 = event-data() -> ()  [unwired: 1 in, 1 out]
        n178 = local read "Stimuli Type"() -> (w327:T1)
        n179 = case shown="\"Vibrotactile\"" w327 {
          tunnel: w334 -> [w336 w340 w344]
          tunnel: w333 -> [w335 w339 w343]
          tunnel: [w336 w340 w344] -> w326
          tunnel: [w335 w339 w343] -> w324
          frame "Transient", Default {
            w337 = T2."Disabled and Grayed Out" ("Disabled")
            w338 = T2."Enabled" ("Disabled")
            n180 = property on="Inter-Stimulus Interval" class="DigNum (strict)"("DisabledEnum"=w338) -> ()  [unwired: 2 in, 2 out]
            n181 = property on="Jitter" class="DigNum (strict)"("DisabledEnum"=w338) -> ()  [unwired: 2 in, 2 out]
            n182 = property on="SSF2" class="DigNum (strict)"("DisabledEnum"=w337) -> ()  [unwired: 2 in, 2 out]
            n183 = property on="SSF3" class="DigNum (strict)"("DisabledEnum"=w337) -> ()  [unwired: 2 in, 2 out]
            n184 = property on="SSF4" class="DigNum (strict)"("DisabledEnum"=w337) -> ()  [unwired: 2 in, 2 out]
            n185 = property on="SSF1" class="DigNum (strict)"("DisabledEnum"=w337) -> ()  [unwired: 2 in, 2 out]
            n186 = property on="SSF5" class="DigNum (strict)"("DisabledEnum"=w337) -> ()  [unwired: 2 in, 2 out]
          }
          frame "Steady State" {
            w341 = T2."Enabled" ("Disabled")
            w342 = T2."Disabled and Grayed Out" ("Disabled")
            n187 = property on="Inter-Stimulus Interval" class="DigNum (strict)"("DisabledEnum"=w342) -> ()  [unwired: 2 in, 2 out]
            n188 = property on="Jitter" class="DigNum (strict)"("DisabledEnum"=w342) -> ()  [unwired: 2 in, 2 out]
            n189 = property on="SSF2" class="DigNum (strict)"("DisabledEnum"=w341) -> ()  [unwired: 2 in, 2 out]
            n190 = property on="SSF3" class="DigNum (strict)"("DisabledEnum"=w341) -> ()  [unwired: 2 in, 2 out]
            n191 = property on="SSF4" class="DigNum (strict)"("DisabledEnum"=w341) -> ()  [unwired: 2 in, 2 out]
            n192 = property on="SSF1" class="DigNum (strict)"("DisabledEnum"=w341) -> ()  [unwired: 2 in, 2 out]
            n193 = property on="SSF5" class="DigNum (strict)"("DisabledEnum"=w341) -> ()  [unwired: 2 in, 2 out]
          }
          frame "Vibrotactile" {
            w345 = T2."Enabled" ("Disabled")
            w346 = T2."Enabled" ("Disabled")
            n194 = property on="Inter-Stimulus Interval" class="DigNum (strict)"("DisabledEnum"=w346) -> ()  [unwired: 2 in, 2 out]
            n195 = property on="Jitter" class="DigNum (strict)"("DisabledEnum"=w346) -> ()  [unwired: 2 in, 2 out]
            n196 = property on="SSF2" class="DigNum (strict)"("DisabledEnum"=w345) -> ()  [unwired: 2 in, 2 out]
            n197 = property on="SSF3" class="DigNum (strict)"("DisabledEnum"=w345) -> ()  [unwired: 2 in, 2 out]
            n198 = property on="SSF4" class="DigNum (strict)"("DisabledEnum"=w345) -> ()  [unwired: 2 in, 2 out]
            n199 = property on="SSF1" class="DigNum (strict)"("DisabledEnum"=w345) -> ()  [unwired: 2 in, 2 out]
            n200 = property on="SSF5" class="DigNum (strict)"("DisabledEnum"=w345) -> ()  [unwired: 2 in, 2 out]
          }
        }
        n201 = Format Into String(format string="%d", initial string="M", w327) -> (resulting string=w328:string)  [unwired: 1 in, 1 out]
        n202 = Concatenate Strings(w328, "\r\n") -> (w329:string)
        n203 = VISA Write(VISA resource name=w326, write buffer=w329, error in (no error)=w324) -> (VISA resource name out=w325:refnum<visa-resource-name>, error out=w323:errorcluster)  [unwired: 1 out]
      }
      event "Cell1": Value Change {
        n204 = event-data() -> ()  [unwired: 1 in, 1 out]
        n205 = Boolean To (0,1)(Boolean="Cell1") -> (0, 1=w357:i16)
        n206 = Format Into String(format string="%1d", initial string="A1", w357) -> (resulting string=w350:string)  [unwired: 1 in, 1 out]
        n207 = Concatenate Strings(w350, "\r\n") -> (w352:string)
        n208 = VISA Write(VISA resource name=w351, write buffer=w352, error in (no error)=w349) -> (VISA resource name out=w347:refnum<visa-resource-name>, error out=w348:errorcluster)  [unwired: 1 out]
      }
      event "Cell2": Value Change {
        n209 = event-data() -> ()  [unwired: 1 in, 1 out]
        n210 = Boolean To (0,1)(Boolean="Cell2") -> (0, 1=w368:i16)
        n211 = Format Into String(format string="%1d", initial string="A2", w368) -> (resulting string=w362:string)  [unwired: 1 in, 1 out]
        n212 = Concatenate Strings(w362, "\r\n") -> (w364:string)
        n213 = VISA Write(VISA resource name=w363, write buffer=w364, error in (no error)=w361) -> (VISA resource name out=w359:refnum<visa-resource-name>, error out=w360:errorcluster)  [unwired: 1 out]
      }
      event "Cell3": Value Change {
        n214 = event-data() -> ()  [unwired: 1 in, 1 out]
        n215 = Boolean To (0,1)(Boolean="Cell3") -> (0, 1=w379:i16)
        n216 = Format Into String(format string="%1d", initial string="A3", w379) -> (resulting string=w373:string)  [unwired: 1 in, 1 out]
        n217 = Concatenate Strings(w373, "\r\n") -> (w375:string)
        n218 = VISA Write(VISA resource name=w374, write buffer=w375, error in (no error)=w372) -> (VISA resource name out=w370:refnum<visa-resource-name>, error out=w371:errorcluster)  [unwired: 1 out]
      }
      event "Cell4": Value Change {
        n219 = event-data() -> ()  [unwired: 1 in, 1 out]
        n220 = Boolean To (0,1)(Boolean="Cell4") -> (0, 1=w390:i16)
        n221 = Format Into String(format string="%1d", initial string="A4", w390) -> (resulting string=w384:string)  [unwired: 1 in, 1 out]
        n222 = Concatenate Strings(w384, "\r\n") -> (w386:string)
        n223 = VISA Write(VISA resource name=w385, write buffer=w386, error in (no error)=w383) -> (VISA resource name out=w381:refnum<visa-resource-name>, error out=w382:errorcluster)  [unwired: 1 out]
      }
      event "Cell5": Value Change {
        n224 = event-data() -> ()  [unwired: 1 in, 1 out]
        n225 = Boolean To (0,1)(Boolean="Cell5") -> (0, 1=w401:i16)
        n226 = Format Into String(format string="%1d", initial string="A5", w401) -> (resulting string=w395:string)  [unwired: 1 in, 1 out]
        n227 = Concatenate Strings(w395, "\r\n") -> (w397:string)
        n228 = VISA Write(VISA resource name=w396, write buffer=w397, error in (no error)=w394) -> (VISA resource name out=w392:refnum<visa-resource-name>, error out=w393:errorcluster)  [unwired: 1 out]
      }
      event "Switch": Value Change {
        n229 = event-data() -> ()  [unwired: 1 in, 1 out]
        n230 = case shown="True" "Switch" {
          tunnel: w406 -> [w412 w419]
          tunnel: [w410 w417] -> w405
          tunnel: w404 -> [w413 w420]
          tunnel: [w411 w418] -> w403
          frame False {
            # "STOP"
            n231 = Concatenate Strings("2" ("write buffer"), "\r\n") -> (w407:string)
            n232 = VISA Write(VISA resource name=w413, write buffer=w407, error in (no error)=w412) -> (VISA resource name out=w411:refnum<visa-resource-name>, error out=w410:errorcluster)  [unwired: 1 out]
          }
          frame True {
            # "START"
            n233 = Concatenate Strings("1" ("write buffer"), "\r\n") -> (w414:string)
            n234 = VISA Write(VISA resource name=w420, write buffer=w414, error in (no error)=w419) -> (VISA resource name out=w418:refnum<visa-resource-name>, error out=w417:errorcluster)  [unwired: 1 out]
          }
        }
      }
      event "Refresh": Value Change {
        n235 = event-data() -> ()  [unwired: 1 in, 1 out]
        n236 = case shown="True" "Refresh" {
          tunnel: w425 -> [w427 w431]
          tunnel: [w427 w430] -> w424
          tunnel: w423 -> [w426 w429]
          tunnel: [w426 w428] -> w422
          frame False {
          }
          frame True {
            n237 = Concatenate Strings("Q" ("write buffer"), "\r\n") -> (w434:string)
            n238 = VISA Write(VISA resource name=w431, write buffer=w434, error in (no error)=w429) -> (VISA resource name out=w430:refnum<visa-resource-name>, error out=w428:errorcluster)  [unwired: 1 out]
          }
        }
      }
    }
  }
  n239 = VISA Close(VISA resource name=w2, error in (no error)=w3) -> (error out=w4:errorcluster)
  n240 = call <vilib>:"Clear Errors.vi"("error in (no error)"=w4) -> ()  [unwired: 6 in, 1 out]
